vi "frontPanel.vi"(8 "error in (no error)":errorcluster, 10 "ScriptEvent":refnum<class "ScriptEvent.lvclass">, 11 "ActionPanel in":refnum<class "SingleToneAction.lvclass">) -> (0 "error out":errorcluster, 2 "ScriptEvent out":refnum<class "ScriptEvent.lvclass">, 3 "SingleToneAction out":refnum<class "SingleToneAction.lvclass">)   [LabVIEW 2011, in "Views.lvlib" / "ScriptEditor.lvlib" / "SingleToneAction.lvclass"]
uses:
  SingleToneAction.lvclass
  Tools/Scripting/ScriptingEvent/ScriptEvent.lvclass
  SingleToneAction.lvclass/SingleToneAction.ctl
  Tools/Scripting/ScriptingEvent/ScriptEvents/SingleTone/SingleTone.lvclass
  Tools/Scripting/ScriptingEvent/ScriptEvents/SingleToneArray/SingleToneArray.lvclass
  ActionPanel.lvclass
panel:
  in  "Current Phase (Degrees)":dbl format="%#.6g"
  in  "Phase (Degrees)":dbl format="%#.6g"
  out "editing":bool
  out "ready?":bool
  in  "close":bool
  in  "Frequency":dbl format="%#.6g"
  in  "States":u16(ring)
  in  "Amplitude":string
  in  "Dt":dbl format="%.6g"
  in  "Time":dbl format="%.6g"
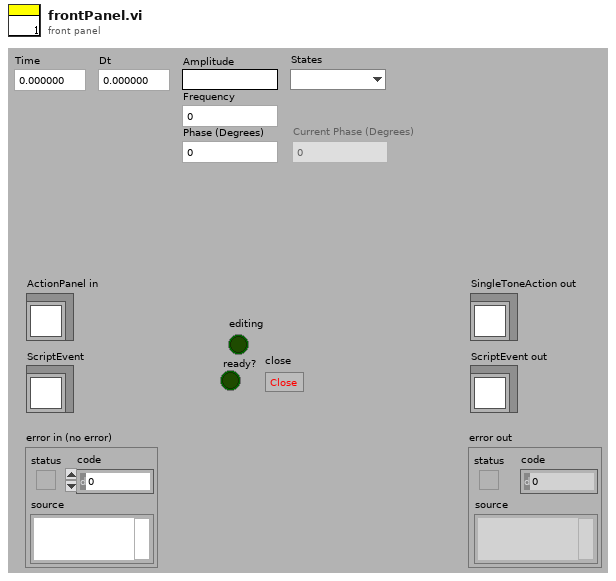
[diagram p1: front panel]
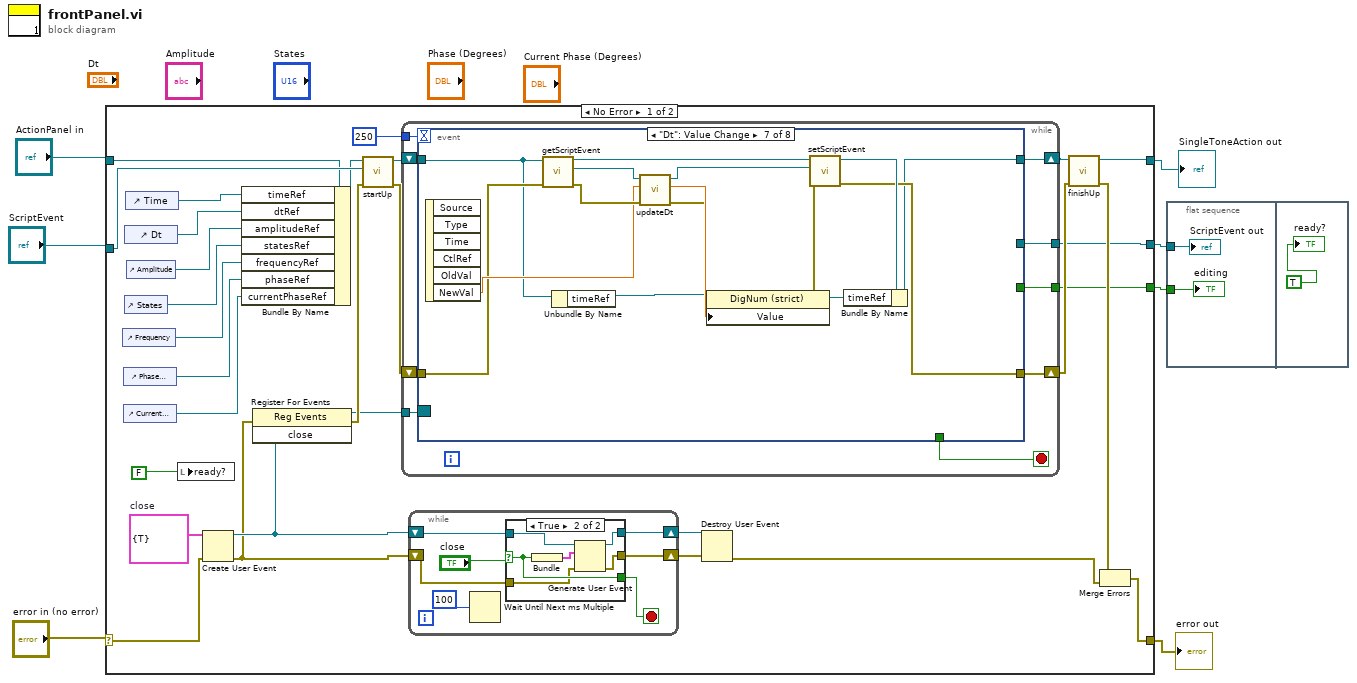
[diagram p0: block diagram]
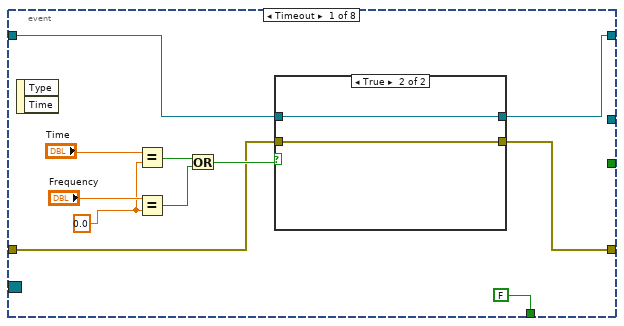
[diagram p3: hidden frame]
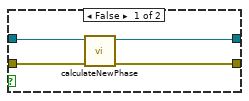
[diagram p4: hidden frame]
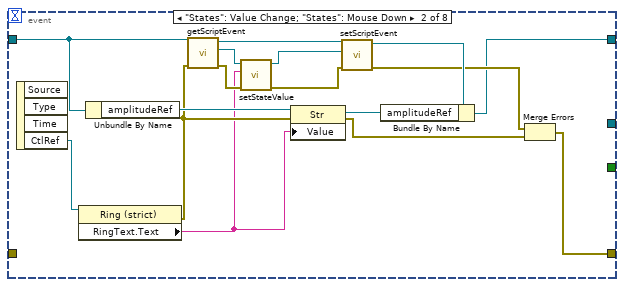
[diagram p5: hidden frame]
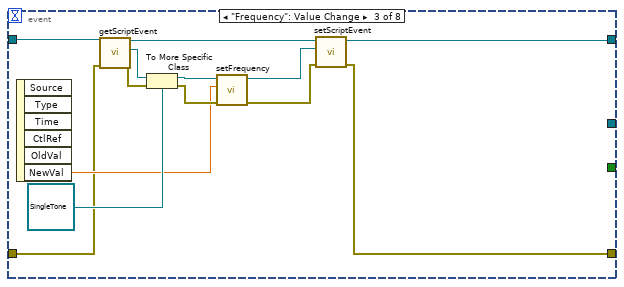
[diagram p6: hidden frame]
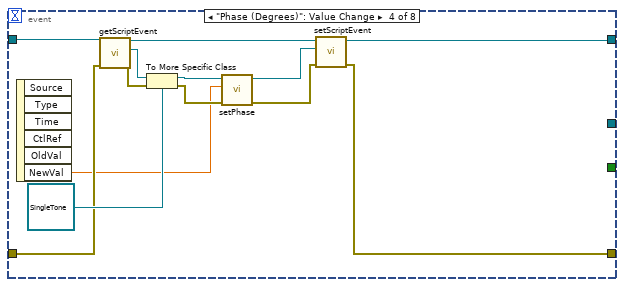
[diagram p7: hidden frame]
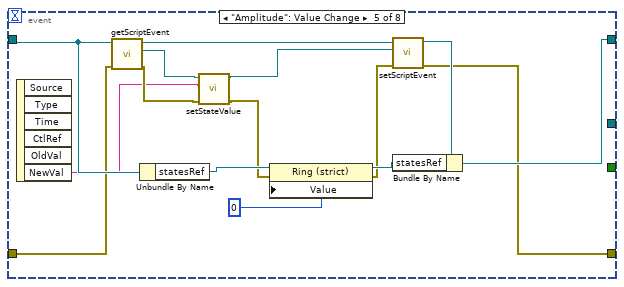
[diagram p8: hidden frame]
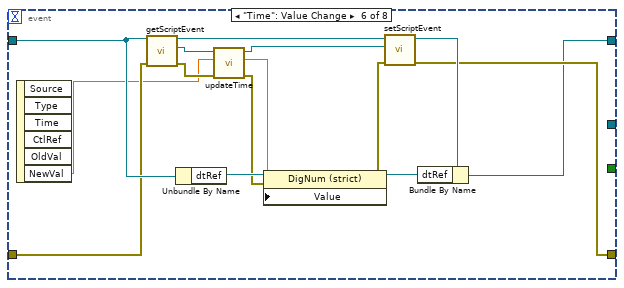
[diagram p9: hidden frame]
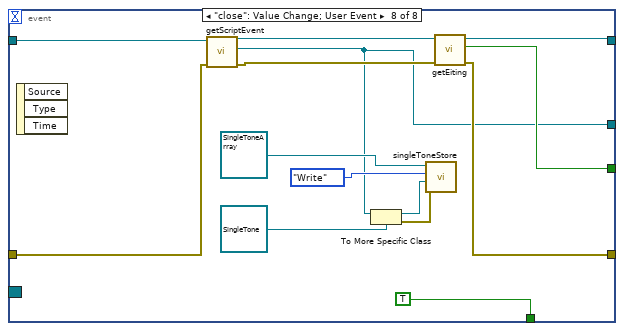
[diagram p10: hidden frame]
diagram:
  n1 = case shown="No Error" "error in (no error)" {
    selector: "error in (no error)" -> [w25 w181]
    tunnel: [w27 w181] -> w6
    tunnel: "ActionPanel in" -> [w17 w183]
    tunnel: [w37 w183] -> w4
    tunnel: "ScriptEvent" -> [w32 w182]
    tunnel: [w19 w182] -> w2
    tunnel: [w18 _] -> w1
    frame No Error {
      w26 = cluster{"close":bool} {"close"=TRUE}  # close
      n2 = control-ref of="Frequency"() -> (w10:refnum<vi>)
      n3 = control-ref of="Phase (Degrees)"() -> (w12:refnum<vi>)
      n4 = control-ref of="Current Phase (Degrees)"() -> (w9:refnum<vi>)
      n5 = control-ref of="Dt"() -> (w13:refnum<vi>)
      n6 = control-ref of="States"() -> (w11:refnum<vi>)
      n7 = control-ref of="Time"() -> (w15:refnum<vi>)
      n8 = control-ref of="Amplitude"() -> (w14:refnum<vi>)
      n9 = local write "ready?"(FALSE) -> ()
      n10 = Create User Event(user event datatype=w26, error in=w25) -> (user event=w24:refnum<user-event>, error out=w23:errorcluster)
      n11 = Bundle By Name(cluster=w17, "timeRef"=w15, "dtRef"=w13, "amplitudeRef"=w14, "statesRef"=w11, "frequencyRef"=w10, "phaseRef"=w12, "currentPhaseRef"=w9) -> (w16:refnum<class "SingleToneAction.lvclass">)
      n12 = register-events(error in=w23, w24) -> (reference out=w21:refnum<event-registration>, error out=w22:errorcluster)  [unwired: 1 in]
      n13 = call-dynamic "startUp.vi"("error in (no error)"=w22, "ScriptEvent"=w32, "SingleToneAction in"=w16) -> ("error out"=w34:errorcluster, "SingleToneAction out"=w35:refnum<class "SingleToneAction.lvclass">)  [unwired: 7 in]
      n14 = while {
        shift-right: [w62] -> w36
        shift-left: w35 -> [w61]
        shift-right: [w59] -> w33
        shift-left: w34 -> [w60]
        tunnel: w21 -> [w57]
        tunnel: [w56] -> w19
        tunnel: [w55] -> w18
        tunnel: 250 -> [w54]
        stop <- w58 stop-if-true
        n15 = event shown="[6] \"Dt\": Value Change" {
          selector: w57 -> [_ _ _ _ _ _ _ _]
          dyn-events: _ -> [_ _ _ _ _ _ _ _]
          timeout: w54 -> [_ _ _ _ _ _ _ _]
          tunnel: [w65 w82 w96 w114 w123 w139 w156 w177] -> w62
          tunnel: w61 -> [w66 w83 w107 w120 w126 w143 w153 w178]
          tunnel: w60 -> [w64 _ w101 w117 w124 w142 w154 w175]
          tunnel: [w63 w81 w97 w115 w122 w140 w157 w176] -> w59
          tunnel: [FALSE _ _ _ _ _ _ TRUE] -> w58
          tunnel: [_ _ _ _ _ _ _ w169] -> w56
          tunnel: [_ _ _ _ _ _ _ w174] -> w55
          event Timeout {
            w70 = 0.0
            n16 = event-data() -> ()  [unwired: 1 in, 2 out]
            n17 = Equal?(x="Time", y=w70) -> (x = y?=w69:bool)
            n18 = Equal?(x="Frequency", y=w70) -> (x = y?=w68:bool)
            n19 = Or(x=w69, y=w68) -> (x .or. y?=w67:bool)
            n20 = case shown="True" w67 {
              tunnel: w66 -> [w77 w79]
              tunnel: [w76 w79] -> w65
              tunnel: w64 -> [w75 w78]
              tunnel: [w74 w78] -> w63
              frame False {
                n21 = call "calculateNewPhase.vi"("error in (no error)"=w75, "SingleToneAction in"=w77) -> ("error out"=w74:errorcluster, "SingleToneAction out"=w76:refnum<class "SingleToneAction.lvclass">)  [unwired: 8 in]
              }
              frame True {
              }
            }
          }
          event "States": Value Change; "States": Mouse Down {
            n22 = event-data() -> ("CtlRef"=w80:refnum<vi>)  [unwired: 1 in, 3 out]
            n23 = property class="Ring (strict)"(reference=w80) -> (error out=w91:errorcluster, "RingText.Text"=w90:string)  [unwired: 1 in, 1 out]
            n24 = Unbundle By Name(w83) -> ("amplitudeRef"=w92:refnum<vi>)
            n25 = call "getScriptEvent.vi"("error in (no error)"=w91, "ActionPanel.lvclass in"=w83) -> ("error out"=w93:errorcluster, "ScriptEvent.lvclass"=w94:refnum<class "ScriptEvent.lvclass">, "ActionPanel.lvclass out"=w95:refnum<class "SingleToneAction.lvclass">)  [unwired: 7 in]
            n26 = call "setStateValue.vi"("error in (no error)"=w93, "stateValue"=w90, "ScriptEvent in"=w94) -> ("error out"=w84:errorcluster, "ScriptEvent out"=w85:refnum<class "ScriptEvent.lvclass">)  [unwired: 7 in]
            n27 = property class="Str"(reference=w92, error in=w91, "Value"=w90) -> (reference out=w89:refnum<vi>, error out=w86:errorcluster)
            n28 = call "setScriptEvent.vi"("error in (no error)"=w84, "ScriptEvent.lvclass"=w85, "ActionPanel.lvclass in"=w95) -> ("error out"=w87:errorcluster, "ActionPanel.lvclass out"=w88:refnum<class "SingleToneAction.lvclass">)  [unwired: 7 in]
            n29 = Bundle By Name(cluster=w88, "amplitudeRef"=w89) -> (w82:refnum<class "SingleToneAction.lvclass">)
            n30 = Merge Errors(w87, w86) -> (w81:errorcluster)
          }
          event "Frequency": Value Change {
            n31 = event-data() -> ("NewVal"=w103:dbl)  [unwired: 1 in, 5 out]
            n32 = call "getScriptEvent.vi"("error in (no error)"=w101, "ActionPanel.lvclass in"=w107) -> ("error out"=w102:errorcluster, "ScriptEvent.lvclass"=w106:refnum<class "ScriptEvent.lvclass">, "ActionPanel.lvclass out"=w100:refnum<class "SingleToneAction.lvclass">)  [unwired: 7 in]
            n33 = To More Specific Class(target class=refnum<class "SingleTone.lvclass"> refnum ("Tools.lvlib:Scripting.lvlib:SingleTone.lvclass"), reference=w106, error in=w102) -> (specific class reference=w105:refnum<class "SingleTone.lvclass">, error out=w104:errorcluster)
            n34 = call "setFrequency.vi"("error in (no error)"=w104, "frequency"=w103, "SingleTone.lvclass in"=w105) -> ("error out"=w98:errorcluster, "SingleTone.lvclass out"=w99:refnum<class "SingleTone.lvclass">)  [unwired: 7 in]
            n35 = call "setScriptEvent.vi"("error in (no error)"=w98, "ScriptEvent.lvclass"=w99, "ActionPanel.lvclass in"=w100) -> ("error out"=w97:errorcluster, "ActionPanel.lvclass out"=w96:refnum<class "SingleToneAction.lvclass">)  [unwired: 7 in]
          }
          event "Phase (Degrees)": Value Change {
            n36 = event-data() -> ("NewVal"=w109:dbl)  [unwired: 1 in, 5 out]
            n37 = call "getScriptEvent.vi"("error in (no error)"=w117, "ActionPanel.lvclass in"=w120) -> ("error out"=w118:errorcluster, "ScriptEvent.lvclass"=w119:refnum<class "ScriptEvent.lvclass">, "ActionPanel.lvclass out"=w116:refnum<class "SingleToneAction.lvclass">)  [unwired: 7 in]
            n38 = To More Specific Class(target class=refnum<class "SingleTone.lvclass"> refnum ("Tools.lvlib:Scripting.lvlib:SingleTone.lvclass"), reference=w119, error in=w118) -> (specific class reference=w113:refnum<class "SingleTone.lvclass">, error out=w110:errorcluster)
            n39 = call "setPhase.vi"("error in (no error)"=w110, "phase"=w109, "SingleTone.lvclass in"=w113) -> ("error out"=w111:errorcluster, "SingleTone.lvclass out"=w112:refnum<class "SingleTone.lvclass">)  [unwired: 7 in]
            n40 = call "setScriptEvent.vi"("error in (no error)"=w111, "ScriptEvent.lvclass"=w112, "ActionPanel.lvclass in"=w116) -> ("error out"=w115:errorcluster, "ActionPanel.lvclass out"=w114:refnum<class "SingleToneAction.lvclass">)  [unwired: 7 in]
          }
          event "Amplitude": Value Change {
            n41 = event-data() -> ("NewVal"=w125:string)  [unwired: 1 in, 5 out]
            n42 = call "getScriptEvent.vi"("error in (no error)"=w124, "ActionPanel.lvclass in"=w126) -> ("error out"=w128:errorcluster, "ScriptEvent.lvclass"=w130:refnum<class "ScriptEvent.lvclass">, "ActionPanel.lvclass out"=w136:refnum<class "SingleToneAction.lvclass">)  [unwired: 7 in]
            n43 = Unbundle By Name(w126) -> ("statesRef"=w135:refnum<vi>)
            n44 = call "setStateValue.vi"("error in (no error)"=w128, "stateValue"=w125, "ScriptEvent in"=w130) -> ("error out"=w127:errorcluster, "ScriptEvent out"=w129:refnum<class "ScriptEvent.lvclass">)  [unwired: 7 in]
            n45 = property class="Ring (strict)"(reference=w135, error in=w127, "Value"=0) -> (reference out=w132:refnum<vi>, error out=w131:errorcluster)
            n46 = call "setScriptEvent.vi"("error in (no error)"=w131, "ScriptEvent.lvclass"=w129, "ActionPanel.lvclass in"=w136) -> ("error out"=w122:errorcluster, "ActionPanel.lvclass out"=w133:refnum<class "SingleToneAction.lvclass">)  [unwired: 7 in]
            n47 = Bundle By Name(cluster=w133, "statesRef"=w132) -> (w123:refnum<class "SingleToneAction.lvclass">)
          }
          event "Time": Value Change {
            n48 = event-data() -> ("NewVal"=w141:dbl)  [unwired: 1 in, 5 out]
            n49 = call "getScriptEvent.vi"("error in (no error)"=w142, "ActionPanel.lvclass in"=w143) -> ("error out"=w149:errorcluster, "ScriptEvent.lvclass"=w150:refnum<class "ScriptEvent.lvclass">, "ActionPanel.lvclass out"=w151:refnum<class "SingleToneAction.lvclass">)  [unwired: 7 in]
            n50 = Unbundle By Name(w143) -> ("dtRef"=w148:refnum<vi>)
            n51 = call "updateTime.vi"("error in (no error)"=w149, "time"=w141, "ScriptEvent in"=w150) -> ("error out"=w137:errorcluster, "dt"=w147:dbl, "ScriptEvent out"=w138:refnum<class "ScriptEvent.lvclass">)  [unwired: 6 in]
            n52 = property class="DigNum (strict)"(reference=w148, error in=w137, "Value"=w147) -> (reference out=w146:refnum<vi>, error out=w144:errorcluster)
            n53 = call "setScriptEvent.vi"("error in (no error)"=w144, "ScriptEvent.lvclass"=w138, "ActionPanel.lvclass in"=w151) -> ("error out"=w140:errorcluster, "ActionPanel.lvclass out"=w145:refnum<class "SingleToneAction.lvclass">)  [unwired: 7 in]
            n54 = Bundle By Name(cluster=w145, "dtRef"=w146) -> (w139:refnum<class "SingleToneAction.lvclass">)
          }
          event "Dt": Value Change {
            n55 = event-data() -> ("NewVal"=w155:dbl)  [unwired: 1 in, 5 out]
            n56 = call "getScriptEvent.vi"("error in (no error)"=w154, "ActionPanel.lvclass in"=w153) -> ("error out"=w161:errorcluster, "ScriptEvent.lvclass"=w162:refnum<class "ScriptEvent.lvclass">, "ActionPanel.lvclass out"=w166:refnum<class "SingleToneAction.lvclass">)  [unwired: 7 in]
            n57 = Unbundle By Name(w153) -> ("timeRef"=w152:refnum<vi>)
            n58 = call "updateDt.vi"("error in (no error)"=w161, "dt"=w155, "ScriptEvent in"=w162) -> ("error out"=w159:errorcluster, "time"=w160:dbl, "ScriptEvent out"=w158:refnum<class "ScriptEvent.lvclass">)  [unwired: 6 in]
            n59 = property class="DigNum (strict)"(reference=w152, error in=w159, "Value"=w160) -> (reference out=w165:refnum<vi>, error out=w163:errorcluster)
            n60 = call "setScriptEvent.vi"("error in (no error)"=w163, "ScriptEvent.lvclass"=w158, "ActionPanel.lvclass in"=w166) -> ("error out"=w157:errorcluster, "ActionPanel.lvclass out"=w164:refnum<class "SingleToneAction.lvclass">)  [unwired: 7 in]
            n61 = Bundle By Name(cluster=w164, "timeRef"=w165) -> (w156:refnum<class "SingleToneAction.lvclass">)
          }
          event "close": Value Change; User Event {
            n62 = event-data() -> ()  [unwired: 1 in, 3 out]
            n63 = call "getScriptEvent.vi"("error in (no error)"=w175, "ActionPanel.lvclass in"=w178) -> ("error out"=w179:errorcluster, "ScriptEvent.lvclass"=w169:refnum<class "ScriptEvent.lvclass">, "ActionPanel.lvclass out"=w180:refnum<class "SingleToneAction.lvclass">)  [unwired: 7 in]
            n64 = To More Specific Class(target class=refnum<class "SingleTone.lvclass"> refnum ("Tools.lvlib:Scripting.lvlib:SingleTone.lvclass"), reference=w169) -> (specific class reference=w167:refnum<class "SingleTone.lvclass">, error out=w170:errorcluster)  [unwired: 1 in]
            n65 = call "singleToneStore.vi"("error in (no error)"=w170, "SingleTone.lvclass"=w167, "action"=enum16{"Write", "Read"}."Write", "SingleToneArray in"=refnum<class "SingleToneArray.lvclass"> refnum) -> ()  [unwired: 4 in, 4 out]
            n66 = call "getEiting.vi"("error in (no error)"=w179, "ActionPanel.lvclass in"=w180) -> ("error out"=w176:errorcluster, "editing?"=w174:bool, "ActionPanel.lvclass out"=w177:refnum<class "SingleToneAction.lvclass">)  [unwired: 7 in]
          }
        }
      }
      n67 = while {
        shift-right: [w41] -> w30
        shift-left: w23 -> [w40]
        shift-right: [w42] -> w31
        shift-left: w24 -> [w44]
        stop <- w43 stop-if-true
        n68 = Wait Until Next ms Multiple(millisecond multiple=100) -> ()  [unwired: 1 out]
        n69 = case shown="True" "close" {
          selector: "close" -> [w47 w51]
          tunnel: w44 -> [w46 w53]
          tunnel: [w47 w51] -> w43
          tunnel: [w46 w50] -> w42
          tunnel: [w45 w49] -> w41
          tunnel: w40 -> [w45 w48]
          frame False {
          }
          frame True {
            n70 = Bundle(w51) -> (w52:cluster{bool})  [unwired: 1 in]
            n71 = Generate User Event(user event=w53, event data cluster=w52, error in=w48) -> (user event out=w50:refnum<user-event>, error out=w49:errorcluster)
          }
        }
      }
      n72 = Destroy User Event(user event=w31, error in=w30) -> (error out=w28:errorcluster)
      n73 = call-dynamic "finishUp.vi"("error in (no error)"=w33, "SingleToneAction in"=w36) -> ("error out"=w29:errorcluster, "SingleToneAction out"=w37:refnum<class "SingleToneAction.lvclass">)  [unwired: 8 in]
      n74 = Merge Errors(w29, w28) -> (w27:errorcluster)
    }
    frame Error {
    }
  }
  "error out" <- w6
  "SingleToneAction out" <- w4
  n75 = flat-sequence {
    tunnel: w2 -> [w185]
    tunnel: w1 -> [w184]
    frame #0 {
      "ScriptEvent out" <- w185
      "editing" <- w184
    }
    frame #1 {
      "ready?" <- TRUE
    }
  }
